vi "LVClass_HasoEngine Set Lift Algorithm Enabled.vi"(0 "HasoEngine in":refnum<class "HasoEngine.lvclass">, 5 "LiftAlgorithmEnable":bool, 7 "Wavelenght_nm":sgl=555.0, 11 "error in (no error)":errorcluster) -> (4 "HasoEngine out":refnum<class "HasoEngine.lvclass">, 15 "error out":errorcluster)   [LabVIEW 2020, in "HasoEngine.lvclass"]
doc: "Spots detection algorithm type setter.\n\n--------------------------------------------------------------------------------\n\n<B>HasoEngineIn </B> : HasoEngine object.\n<B>HasoEngineOut </B> : HasoEngine object.\n<B>algo_type </B> : Lift algorithm activation : Enable (T) / disable (F).\n<B>ErrorIn </B> : Error\n<B>ErrorOut </B> : Error\n\n--------------------------------------------------------------------------------"
uses:
  HasoEngine.lvclass
  HasoEngine.lvclass/HasoEngine.ctl
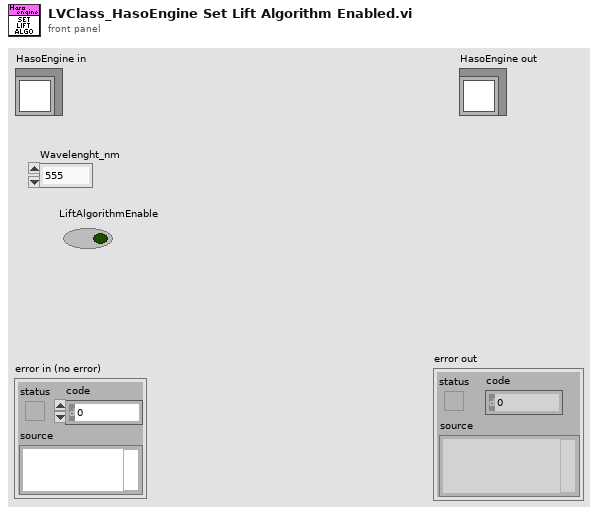
[diagram p1: front panel]
types:
  T1 = typedef "ClassID.ctl" = i64
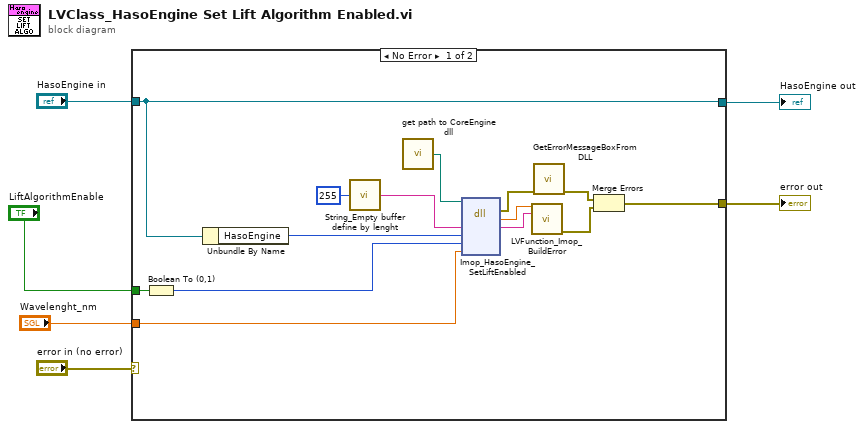
[diagram p0: block diagram]
diagram:
  n1 = case shown="No Error" "error in (no error)" {
    selector: "error in (no error)" -> [_ w21]
    tunnel: "HasoEngine in" -> [w15 w22]
    tunnel: [w15 w22] -> w3
    tunnel: [w10 w21] -> w4
    tunnel: "LiftAlgorithmEnable" -> [w9 _]
    tunnel: "Wavelenght_nm" -> [w7 _]
    frame No Error {
      n2 = Boolean To (0,1)(Boolean=w9) -> (0, 1=w8:i16)
      n3 = Unbundle By Name(w15) -> ("HasoEngine"=w14:T1)
      n4 = call "String_Empty buffer define by lenght.vi"("Lenght (255)"=255) -> ("Empty buffer"=w18:string)
      n5 = call "get path to CoreEngine dll.vi"() -> ("path to wavekit library"=w17:path)  [unwired: 14 in, 1 out]
      n6 = dll-call lib="D:/soft/HASO_v3/SVN_trunk/ImOpCoreEngine4_LV2011/DLLs/c_interface_vc100.dll" fn="Imop_HasoEngine_SetLiftEnabled"(path in=w17, "message"=w18, "hasoEngine"=w14, "enable_spot_tracker"=w8, "Wavelenght_nm"=w7) -> (error out=w16:errorcluster, "return type"=w19:sgl, "message"=w20:string)  [unwired: 5 in, 1 out]
      n7 = call "LVFunction_Imop_BuildError.vi"("code"=w19, "String to Prepend to source (\"\")"=w20) -> ("error out"=w11:errorcluster)  [unwired: 13 in]
      n8 = call "GetErrorMessageBoxFromDLL.vi"("error IN"=w16) -> ("error OUT"=w12:errorcluster)  [unwired: 10 in]
      n9 = Merge Errors(w12, w11) -> (w10:errorcluster)
    }
    frame Error {
    }
  }
  "error out" <- w4
  "HasoEngine out" <- w3
